vi "SHIFTER - TLB` Springboard.vi"() -> (8 "SHIFTER DATA":T1)   [LabVIEW 2015, in "TLB` Springboard.lvlib"]
doc: "TLB Prime - Application Template 1.3.0.24\nNorm Kirchner, NI Systems Engineering - NI\nCopyright (c) 2014, NI"
uses:
  TLB` Springboard.lvlib
  TypeDef - SHIFTER - TLB` Springboard.ctl
  State Declaration.ctl
  Dependencies.llb/Exit Event Ref.ctl
  Dependencies.llb/TLB`_Dependencies.lvlib
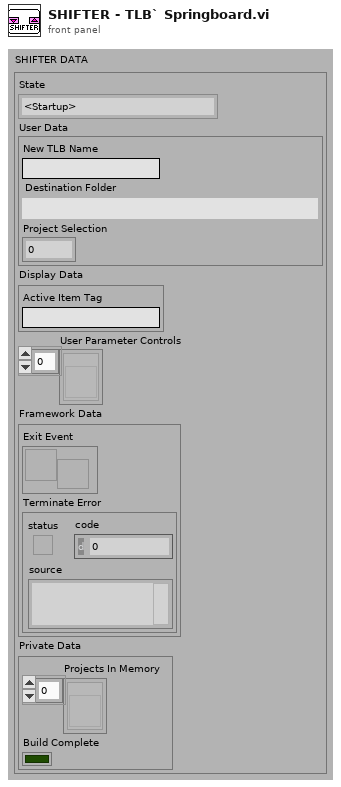
[diagram p1: front panel]
types:
  T1 = typedef "TLB` Springboard.lvlib/TypeDef - SHIFTER - TLB` Springboard.ctl" = cluster{"State":T2, "User Data":cluster{"New TLB Name":string, "Destination Folder":path, "Project Selection":u16}, "Display Data":cluster{"Active Item Tag":string}, "User Parameter Controls":refnum<vi>[], "Framework Data":cluster{"Exit Event":T3, "Terminate Error":errorcluster}, "Private Data":cluster{"Projects In Memory":refnum<vi>[], "Build Complete":bool}}
  T2 = typedef "TLB` Springboard.lvlib/State Declaration.ctl" = enum16{"<Startup>", "Idle", "Creating", "<Shutdown>"}
  T3 = typedef "TLB` Springboard.lvlib/TLB`_Dependencies.lvlib/Exit Event Ref.ctl" = refnum<user-event>
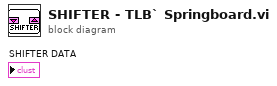
[diagram p0: block diagram]
diagram:
